vi "Read I32.vi"(8 "Error In":errorcluster, 9 "from (0:start)":enum16{"start", "end", "current"}(ring), 10 "offset (in bytes) (0)":i64, 11 "WFM file ref":T1={"refnum"=refnum, "byte order"=enum."little-endian", "Version"=0}) -> (0 "Error Out":errorcluster, 2 "data":i32, 3 "WFM file ref out":T1={"refnum"=refnum, "byte order"=enum."little-endian", "Version"=0})   [LabVIEW 2015]
uses:
  WFM file ref.ctl
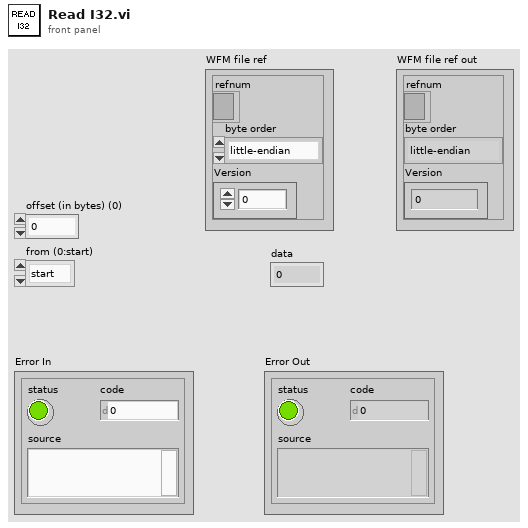
[diagram p1: front panel]
types:
  T1 = typedef "WFM file ref.ctl" = cluster{"refnum":refnum<file>, "byte order":enum16{"big-endian, network order", "native, host order", "little-endian"}, "Version":i32}
  T2 = enum16{"big-endian, network order", "native, host order", "little-endian"}
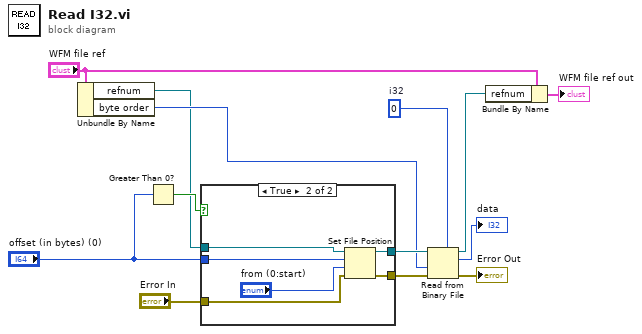
[diagram p0: block diagram]
diagram:
  w12 = 0  # i32
  n1 = Unbundle By Name("WFM file ref") -> ("refnum"=w2:refnum<file>, "byte order"=w3:T2)
  n2 = Greater Than 0?(x="offset (in bytes) (0)") -> (x > 0?=w8:bool)
  n3 = case shown="True" w8 {
    tunnel: w2 -> [w15 w21]
    tunnel: "offset (in bytes) (0)" -> [_ w20]
    tunnel: [w15 w18] -> w13
    tunnel: "Error In" -> [w14 w17]
    tunnel: [w14 w16] -> w10
    frame False {
    }
    frame True {
      n4 = Set File Position(offset (in bytes) (0)=w20, refnum=w21, from (0:start)="from (0:start)", error in=w17) -> (refnum out=w18:refnum<file>, error out=w16:errorcluster)
    }
  }
  n5 = Read from Binary File(5:w12, 8:w10, 9:w3, 11:w13) -> (0:→"Error Out":errorcluster, 2:→"data":i32, 3:w1:refnum<file>)  [unwired: 2 in, 1 out]
  n6 = Bundle By Name(cluster="WFM file ref", "refnum"=w1) -> (→"WFM file ref out":T1)
